vi "test_scd_TriggerModes.vi"(8 "error in":errorcluster, 11 "SCD in":refnum<class "SCD.lvclass">) -> (0 "error out":errorcluster, 3 "SCD out":refnum<class "SCD.lvclass">)   [LabVIEW 2023, in "horiba.test.lvlib"]
uses:
  horiba.test.lvlib
  Classes/SCD/SCD.lvclass
  C:/Projects/Horiba/horiba-labview-sdk/Source/Classes/GenericDevice/GenericDevice.lvclass
  <vilib>/addons/_JKI Toolkits/Caraya/classes/Assert/Assert Equal Value_Variant.vi
  <vilib>/addons/_JKI Toolkits/Caraya/classes/Test/Test.lvclass
  <vilib>/addons/_JKI Toolkits/Caraya/classes/Assert/Assert.lvclass
  <userlib>/_OpenG.lib/lvdata/lvdata.llb/openg_variant.lvlib
panel:
  out "TriggerMode 3":T1
  out "TriggerMode 2":T1
  out "TriggerMode":T1
  # "Connector Pane"
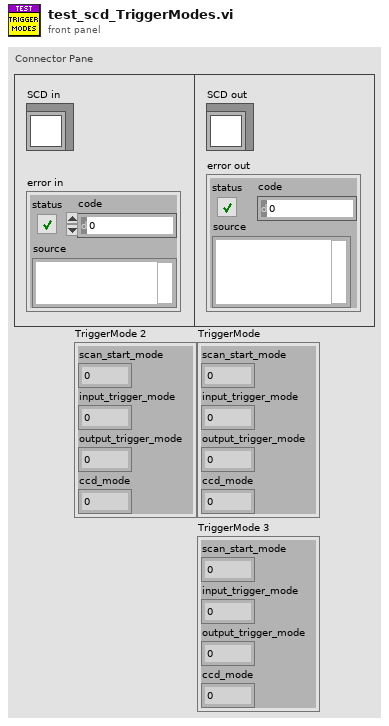
[diagram p1: front panel]
types:
  T1 = cluster{"scan_start_mode":i32, "input_trigger_mode":i32, "output_trigger_mode":i32, "ccd_mode":i32}
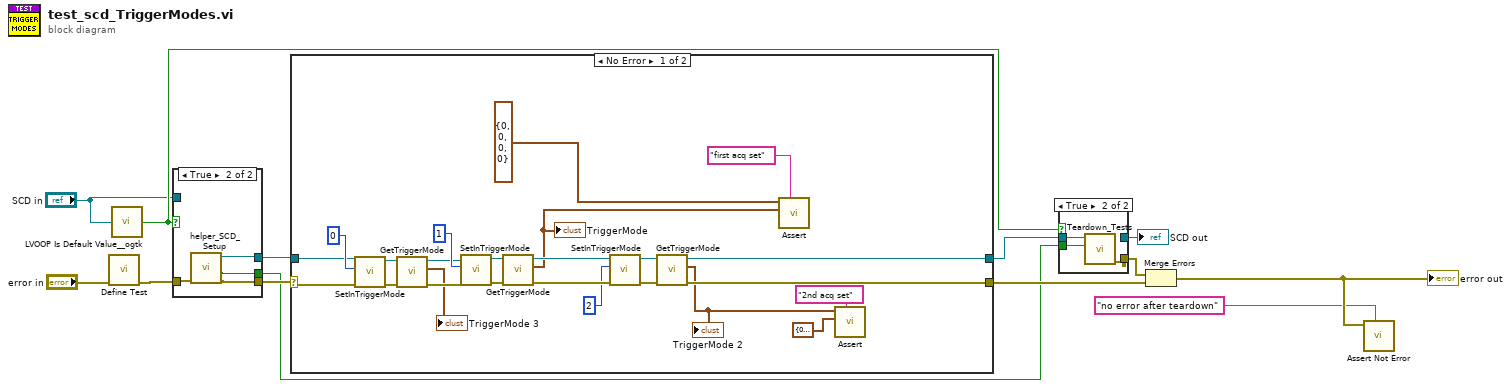
[diagram p0: block diagram]
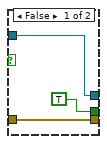
[diagram p3: hidden frame]
diagram:
  n1 = call <vilib>:"Define Test.vi"("error in (no error)"="error in") -> ("error out"=w9:errorcluster)  [unwired: 9 in, 1 out]
  n2 = call <userlib>:"LVOOP Is Default Value__ogtk.vi"("Object"="SCD in") -> ("Is Default Value?"=w3:bool)
  n3 = case shown="True" w3 {
    tunnel: w9 -> [w16 w18]
    tunnel: [w16 w20] -> w8
    tunnel: [w14 w17] -> w7
    tunnel: [TRUE ("Module Was Already Running?") w19] -> w4
    tunnel: "SCD in" -> [w14 _]
    frame False {
    }
    frame True {
      n4 = call "helper_SCD_Setup.vi"("error in"=w18) -> ("error out"=w20:errorcluster, "Module Was Already Running?"=w19:bool, "SCD out"=w17:refnum<class "SCD.lvclass">)  [unwired: 7 in, 1 out]
    }
  }
  n5 = case shown="No Error" w8 {
    selector: w8 -> [w23 w46]
    tunnel: [w36 w45] -> w12
    tunnel: w7 -> [w25 w45]
    tunnel: [w38 w46] -> w11
    frame No Error {
      n6 = call "SetInTriggerMode.vi"("error in (no error)"=w23, "mode"=0, "SCD in"=w25) -> ("error out"=w26:errorcluster, "SCD out"=w27:refnum<class "SCD.lvclass">)  [unwired: 7 in]
      n7 = call "GetTriggerMode.vi"("error in (no error)"=w26, "SCD in"=w27) -> ("error out"=w22:errorcluster, "TriggerMode"=→"TriggerMode 3":T1, "SCD out"=w24:refnum<class "SCD.lvclass">)  [unwired: 7 in]
      n8 = call "SetInTriggerMode.vi"("error in (no error)"=w22, "mode"=1, "SCD in"=w24) -> ("error out"=w43:errorcluster, "SCD out"=w41:refnum<class "SCD.lvclass">)  [unwired: 7 in]
      n9 = call "GetTriggerMode.vi"("error in (no error)"=w43, "SCD in"=w41) -> ("error out"=w42:errorcluster, "TriggerMode"=w33:T1, "SCD out"=w39:refnum<class "SCD.lvclass">)  [unwired: 7 in]
      "TriggerMode" <- w33
      n10 = call "SetInTriggerMode.vi"("error in (no error)"=w42, "mode"=2, "SCD in"=w39) -> ("error out"=w40:errorcluster, "SCD out"=w37:refnum<class "SCD.lvclass">)  [unwired: 7 in]
      n11 = call "GetTriggerMode.vi"("error in (no error)"=w40, "SCD in"=w37) -> ("error out"=w38:errorcluster, "TriggerMode"=w34:T1, "SCD out"=w36:refnum<class "SCD.lvclass">)  [unwired: 7 in]
      "TriggerMode 2" <- w34
      n12 = call-poly <vilib>:"Assert.vi"("Label"="first acq set", "Y"=w33, "X"=T1 {"scan_start_mode"=0, "input_trigger_mode"=0, "output_trigger_mode"=0, "ccd_mode"=0} ("TriggerMode 2")) -> ()  [unwired: 7 in, 2 out]
      n13 = call-poly <vilib>:"Assert.vi"("Label"="2nd acq set", "Y"=T1 {"scan_start_mode"=0, "input_trigger_mode"=0, "output_trigger_mode"=0, "ccd_mode"=0} ("TriggerMode"), "X"=w34) -> ()  [unwired: 7 in, 2 out]
    }
    frame Error {
    }
  }
  n14 = case shown="True" w3 {
    tunnel: w12 -> [w47 w50]
    tunnel: [_ w49] -> w6
    tunnel: w4 -> [_ w48]
    tunnel: [w47 _] -> w1
    frame False {
    }
    frame True {
      n15 = call "Teardown_Tests.vi"("Module Was Already Running?"=w48, "horiba.lvlib:GenericDevice"=w50) -> ("error out"=w49:errorcluster)  [unwired: 8 in, 1 out]
    }
  }
  "SCD out" <- w1
  n16 = Merge Errors(w6, w11) -> (w10:errorcluster)
  "error out" <- w10
  n17 = call <vilib>:"Assert Not Error.vi"("Label"="no error after teardown", "Not Error?"=w10) -> ()  [unwired: 8 in, 2 out]
